vi "dsdll_output_stop.vi"(8 "error in":errorcluster, 11 "dsdll instance in":T1={"dsdll path"=path "E:/LVprog/DirectSoundDLL/dsdll.dll", "dsdll handle"=[], "output devices"=[], "capture devices"=[]}) -> (0 "error out":errorcluster, 3 "dsdll instance out":T1)   [LabVIEW 2020, in "dsdll.lvlib"]
doc: "Call this to stop output device playback."
uses:
  dsdll.lvlib
  dsdll_instance.ctl
  dsdll_device_record.ctl
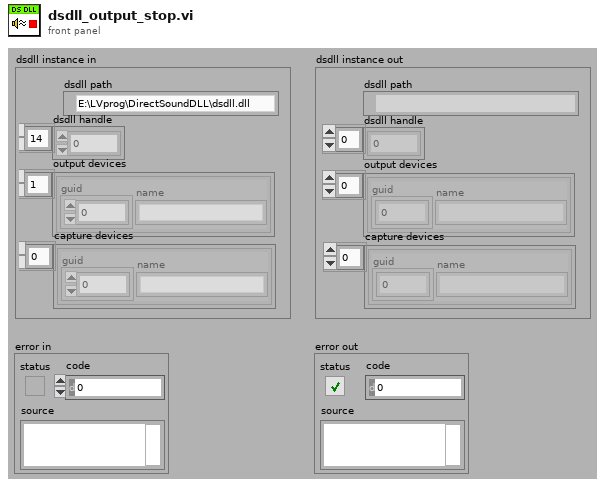
[diagram p1: front panel]
types:
  T1 = typedef "dsdll.lvlib/dsdll_instance.ctl" = cluster{"dsdll path":path, "dsdll handle":u8[], "output devices":T2[], "capture devices":T2[]}
  T2 = typedef "dsdll.lvlib/dsdll_device_record.ctl" = cluster{"guid":u8[], "name":string}
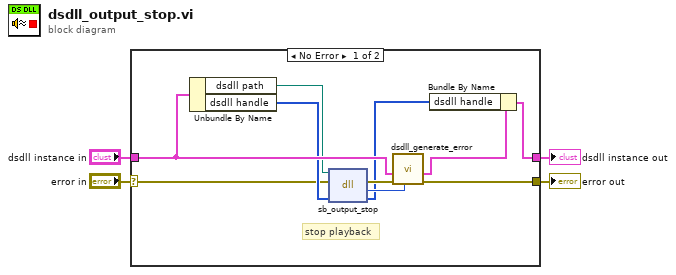
[diagram p0: block diagram]
diagram:
  n1 = case shown="No Error" "error in" {
    selector: "error in" -> [w5 w15]
    tunnel: "dsdll instance in" -> [w12 w16]
    tunnel: [w9 w15] -> w3
    tunnel: [w6 w16] -> w4
    frame No Error {
      # "stop playback"
      n2 = Unbundle By Name(w12) -> ("dsdll path"=w11:path, "dsdll handle"=w10:u8[])
      n3 = dll-call lib="dsdll.dll" fn="sb_output_stop" ("sb_get_handle_size()")(path in=w11, error in=w5, "handle"=w10) -> (error out=w14:errorcluster, "error"=w13:i32, "handle"=w7:u8[])  [unwired: 1 in, 1 out]
      n4 = call "dsdll_generate_error.vi"("error code"=w13, "error in"=w14, "dsdll instance in"=w12) -> ("error out"=w9:errorcluster, "dsdll instance out"=w8:T1)  [unwired: 6 in, 1 out]
      n5 = Bundle By Name(cluster=w8, "dsdll handle"=w7) -> (w6:T1)
    }
    frame Error {
    }
  }
  "error out" <- w3
  "dsdll instance out" <- w4
